vi "Encode COB-ID.vi"(9 "Function code":T1=11 items=["NMT"=0, "EMCY/SYNC"=1, "TIME"=2, "PDO1 (tx)"=3, "PDO1 (rx)"=4, "PDO2 (tx)"=5, "PDO2 (rx)"=6, "PDO3 (tx)"=7, "PDO3 (rx)"=8, "PDO4 (tx)"=9, "PDO4 (rx)"=10, "SDO (tx)"=11, "SDO (rx)"=12, "NMT error control"=14], 11 "Node-ID":u8) -> (3 "COB-ID":u32 format="%.0x")   [LabVIEW 2020, in "CANopen.lvlib" / "CANopen Message.lvclass"]
uses:
  CANopen Message.lvclass
  CANopen Message.lvclass/CANopen Message.ctl
  Typedefs/Function Code.ctl
  CANopen.lvlib
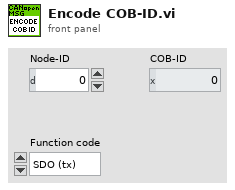
[diagram p1: front panel]
types:
  T1 = typedef "CANopen.lvlib/Function Code.ctl" = u8
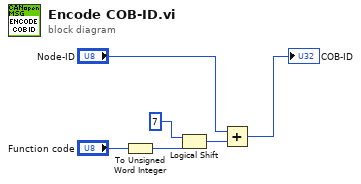
[diagram p0: block diagram]
diagram:
  n1 = To Unsigned Word Integer(number="Function code") -> (unsigned 16bit integer=w1:u16)
  n2 = Logical Shift(y=i16 7, x=w1) -> (x << y=w5:u16)
  n3 = Add(x="Node-ID", y=w5) -> (x+y=→"COB-ID":u16)
